vi "Day1a.vi"() -> ()   [LabVIEW 2019]
uses:
  <vilib>/Utility/file.llb/Read Delimited Spreadsheet (I64).vi
panel:
  out "max value 2":i64
  out "sum 2":i64
  out "sum":i64
  out "max value":i64
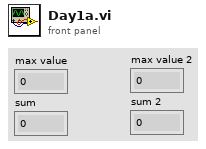
[diagram p1: front panel]
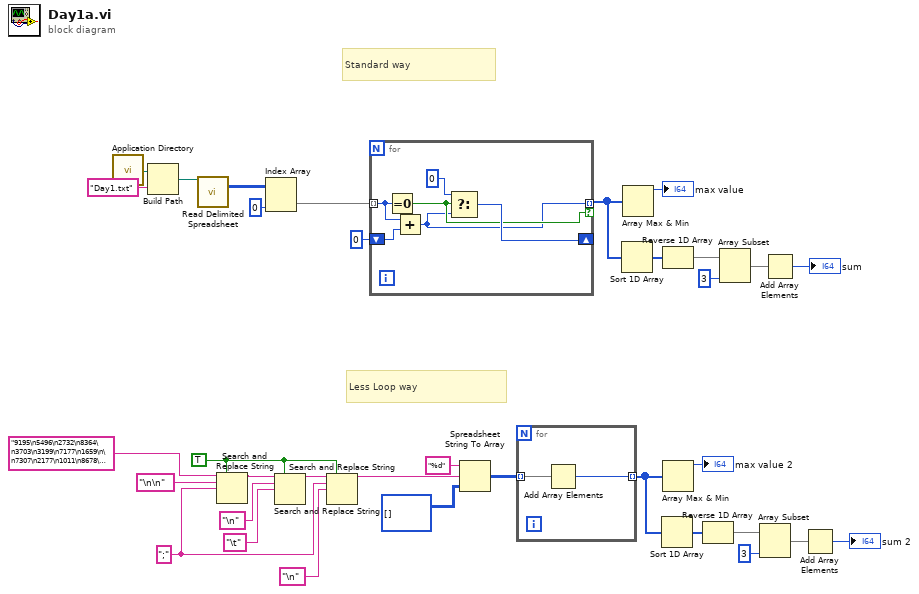
[diagram p0: block diagram]
diagram:
  w10 = ";"
  w12 = TRUE ("replace all? (F)")
  # "Less Loop way"
  # "Standard way"
  n1 = call <vilib>:"Application Directory.vi"() -> ("Application Directory"=w34:path)
  n2 = Build Path(base path=w34, name or relative path="Day1.txt") -> (appended path=w32:path)
  n3 = call-poly <vilib>:"Read Delimited Spreadsheet.vi"("file path (dialog if empty)"=w32) -> ("all rows"=w31:i64[][])  [unwired: 9 in, 5 out]
  n4 = Search and Replace String(replace all?=w12, input string="9195\n5496\n2732\n8364\n3703\n3199\n7177\n1659\n\n7307\n2177\n1011\n8678\n14080\n\n6465\n6922\n3733\n8573\n6749\n1704\n6429\n8774\n1296\n2536\n\n22456\n\n11642\n10162\n10997\n6963\n3076\n5859\n1280\n\n5285\n7498\n8540\n7360\n6822\n8042\n6798\n6398\n4495\n8043\n\n60304\n\n2947\n24880\n21239\n\n8441\n1034\n2591\n8993\n10366\n1313\n10497\n\n3404\n5018\n5377\n4783\n6441\n5110\n5688\n3371\n1220\n4949\n2945\n6041\n2852\n2379\n\n15514\n13699\n10357\n9769\n\n11464\n2001\n2847\n9933\n2706\n8621\n2064\n\n5478\n2981\n6540\n2303\n4607\n5284\n4762\n3936\n3194\n4371\n2925\n3124\n4491\n\n8542\n7605\n3773\n8575\n3405\n4720\n7857\n7427\n5182\n3977\n\n9405\n16048\n4142\n9101\n16303\n\n6102\n1795\n1053\n2091\n5774\n6053\n4997\n2109\n1019...", search string="\n\n" ("regular expression"), replace string=w10) -> (result string=w17:string)  [unwired: 4 in, 3 out]
  n5 = Index Array(array=w31, index (col)=0 ("disabled index (col)")) -> (element=w27:i64[])  [unwired: 1 in]
  n6 = Search and Replace String(replace all?=w12, input string=w17, search string="\n" ("regular expression"), replace string="\t" ("replace string (\"\")")) -> (result string=w14:string)  [unwired: 4 in, 3 out]
  n7 = Search and Replace String(replace all?=w12, input string=w14, search string=w10, replace string="\n" ("regular expression")) -> (result string=w11:string)  [unwired: 4 in, 3 out]
  n8 = for {
    tunnel: w27 -> [w40] mode=indexing
    shift-right: [w37] -> _
    shift-left: i64 0 ("t") -> [w39]
    tunnel: [w35] -> w24 mode=indexing if=w36
    n9 = Equal To 0?(x=w40) -> (x = 0?=w36:bool)
    n10 = Add(x=w40, y=w39) -> (x+y=w35:i64)
    n11 = Select(t=i64 0, s=w36, f=w35) -> (s? t:f=w37:i64)
  }
  n12 = Spreadsheet String To Array(format string="%d", spreadsheet string=w11, array type (2D Dbl)=i32[][] []) -> (array=w8:i32[][])  [unwired: 1 in]
  n13 = for {
    tunnel: w8 -> [w42] mode=indexing
    tunnel: [w41] -> w1 mode=indexing
    n14 = Add Array Elements(numeric array=w42) -> (sum=w41:i32)
  }
  n15 = Sort 1D Array(array=w24) -> (sorted array=w23:i64[])
  n16 = Array Max & Min(array=w24) -> (max value=→"max value":i64)  [unwired: 3 out]
  n17 = Sort 1D Array(array=w1) -> (sorted array=w3:i32[])
  n18 = Reverse 1D Array(array=w23) -> (reversed array=w22:i64[])
  n19 = Array Max & Min(array=w1) -> (max value=→"max value 2":i32)  [unwired: 3 out]
  n20 = Reverse 1D Array(array=w3) -> (reversed array=w4:i32[])
  n21 = Array Subset(array=w22, length=3) -> (w20:i64[])  [unwired: 1 in]
  n22 = Array Subset(array=w4, length=3) -> (w6:i32[])  [unwired: 1 in]
  n23 = Add Array Elements(numeric array=w20) -> (sum=→"sum":i64)
  n24 = Add Array Elements(numeric array=w6) -> (sum=→"sum 2":i32)
